vi "Duplicate.vi"(8 "error in":errorcluster, 10 "parameters":variant, 11 "group in":refnum<class "device.lvclass">) -> (0 "error out":errorcluster, 3 "group copy":refnum<class "device.lvclass">)   [LabVIEW 2013, in "device.lvclass"]
uses:
  device.lvclass
  device registry command.ctl
  device.lvclass/device.ctl
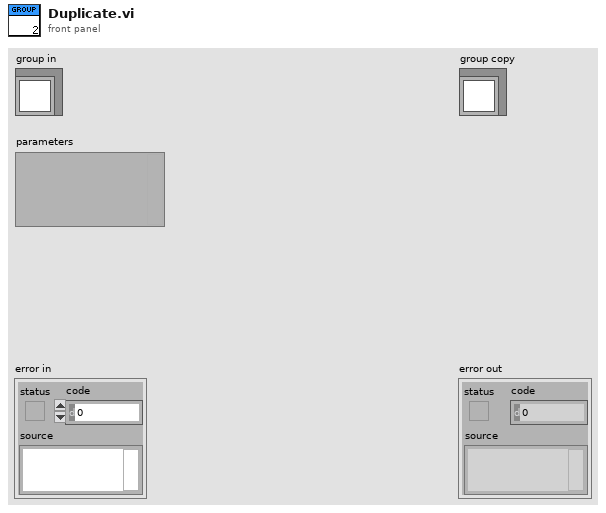
[diagram p1: front panel]
types:
  T1 = typedef "device.lvclass/device registry command.ctl" = enum16{"add device", "remove device", "get next available"}
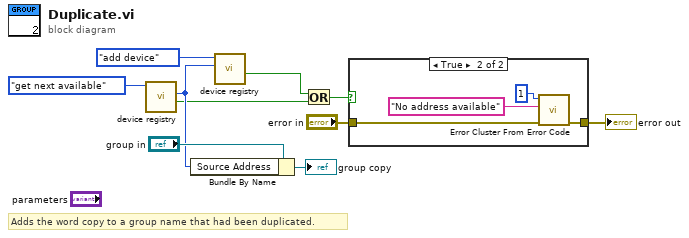
[diagram p0: block diagram]
diagram:
  # "Adds the word copy to a group name that had been duplicated."
  n1 = call "device registry.vi"("command"=device_registry_command."get next available") -> ("Error?"=w4:bool, "device out"=w6:u8)  [unwired: 9 in]
  n2 = Bundle By Name(cluster="group in", "Source Address"=w6) -> (→"group copy":refnum<class "device.lvclass">)
  n3 = call "device registry.vi"("device"=w6, "command"=device_registry_command."add device") -> ("Error?"=w5:bool)  [unwired: 8 in, 1 out]
  n4 = Or(x=w5, y=w4) -> (x .or. y?=w3:bool)
  n5 = case shown="True" w3 {
    tunnel: "error in" -> [w11 w15]
    tunnel: [w11 w14] -> w1
    frame False {
    }
    frame True {
      n6 = call <vilib>:"Error Cluster From Error Code.vi"("error in (no error)"=w15, "error message (\"\")"="No address available" ("error message (\"\")"), "error code (0)"=1) -> ("error out"=w14:errorcluster)  [unwired: 6 in]
    }
  }
  "error out" <- w1
